vi "IKNEW.vi"(8 "L1":dbl=80.0, 10 "L2":dbl=80.0, 11 "Cluster":cluster{"x":dbl, "y":dbl}) -> (1 "theta21":dbl, 2 "theta11":dbl)   [LabVIEW 2024]
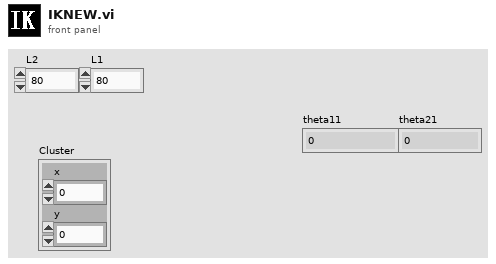
[diagram p1: front panel]
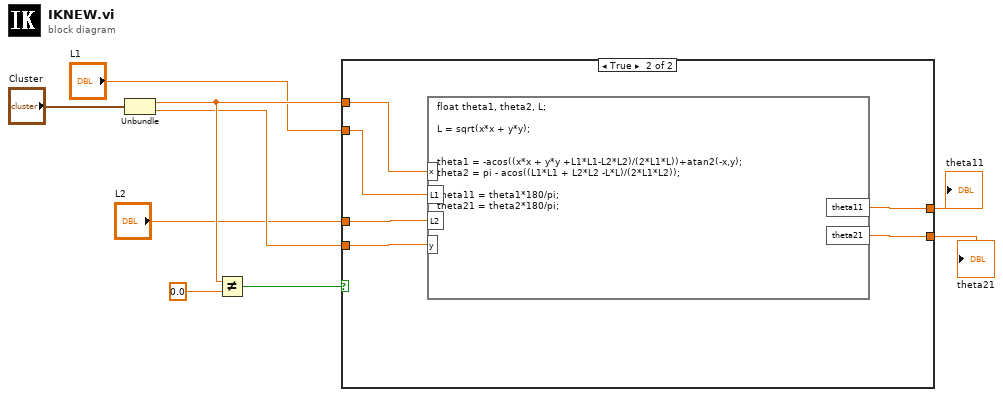
[diagram p0: block diagram]
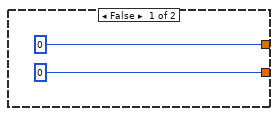
[diagram p2: hidden frame]
diagram:
  n1 = Unbundle("Cluster") -> ("x"=w9:dbl, "y"=w6:dbl)
  n2 = Not Equal?(x=w9, y=0.0) -> (x != y?=w7:bool)
  n3 = case shown="True" w7 {
    tunnel: "L1" -> [_ w17]
    tunnel: "L2" -> [_ w16]
    tunnel: [0 w15] -> w4
    tunnel: [0 w14] -> w3
    tunnel: w9 -> [_ w13]
    tunnel: w6 -> [_ w12]
    frame False {
    }
    frame True {
      n4 = formula code="float theta1, theta2, L;\n\nL = sqrt(x*x + y*y);\n\n\ntheta1 = -acos((x*x + y*y +L1*L1-L2*L2)/(2*L1*L))+atan2(-x,y);\ntheta2 = pi - acos((L1*L1 + L2*L2 -L*L)/(2*L1*L2));\n\ntheta11 = theta1*180/pi;\ntheta21 = theta2*180/pi;"("L1"=w17, "L2"=w16, "x"=w13, "y"=w12) -> ("theta11"=w15:dbl, "theta21"=w14:dbl)
    }
  }
  "theta11" <- w4
  "theta21" <- w3
